vi "Calculate Acquisition Time.vi"(0 "Refnum in":refnum<k21>, 5 "Number of Samples":i32, 11 "error in (no error)":errorcluster) -> (4 "Refnum out":refnum<k21>, 6 "Acquisition Time Period (s)":dbl, 15 "error out":errorcluster)   [LabVIEW 2021]
doc: "This VI is used to calculate the expected acquisition time based on timing details\nAcq Time = No of Samples/Sampling Rate"
uses:
  <resource>/objmgr/daqmx.rc
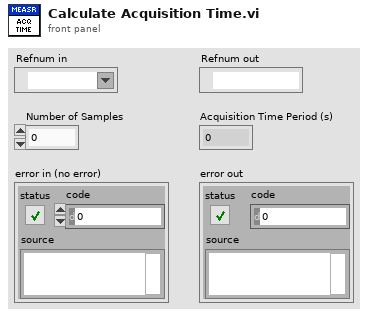
[diagram p1: front panel]
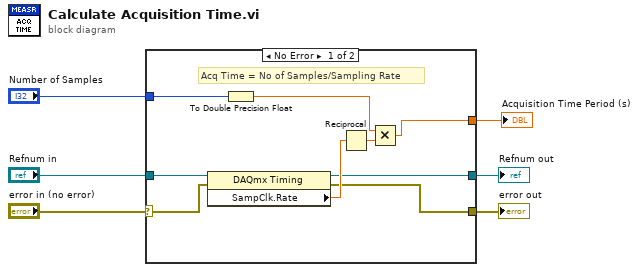
[diagram p0: block diagram]
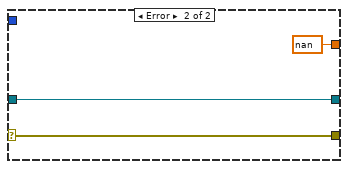
[diagram p2: hidden frame]
diagram:
  n1 = case shown="No Error" "error in (no error)" {
    selector: "error in (no error)" -> [w9 w18]
    tunnel: [w15 nan] -> w6
    tunnel: "Number of Samples" -> [w13 _]
    tunnel: [w11 w17] -> w4
    tunnel: [w10 w18] -> w3
    tunnel: "Refnum in" -> [w8 w17]
    frame No Error {
      # "Acq Time = No of Samples/Sampling Rate"
      n2 = property class="DAQmx Timing"(reference=w8, error in=w9) -> (reference out=w11:refnum<k21>, error out=w10:errorcluster, "SampClk.Rate"=w14:dbl)
      n3 = To Double Precision Float(number=w13) -> (double precision float=w7:dbl)
      n4 = Reciprocal(x=w14) -> (1/x=w12:dbl)
      n5 = Multiply(x=w7, y=w12) -> (x*y=w15:dbl)
    }
    frame Error {
    }
  }
  "Acquisition Time Period (s)" <- w6
  "Refnum out" <- w4
  "error out" <- w3
